vi "Set Comment.vi"(8 "error in (no error)":errorcluster, 10 "Comment":string, 11 "Device in":refnum<class "Device.lvclass">) -> (0 "error out":errorcluster, 3 "Device out":refnum<class "Device.lvclass">)   [LabVIEW 2012, in "HAL.lvlib" / "Device.lvclass"]
uses:
  Device.lvclass
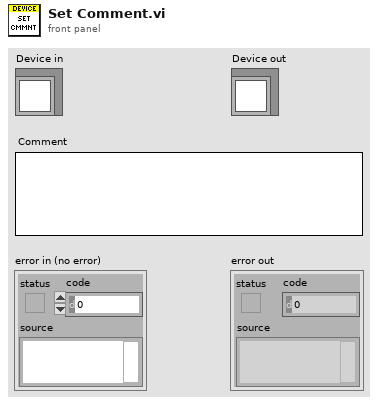
[diagram p1: front panel]
types:
  T1 = typedef "HAL.lvlib/Device.lvclass/Ref Data.ctl" = cluster{"Config Keys":string[], "Config Values":string[], "Cal Expires":timestamp, "Name":string, "Comment":string, "State":T2, "Error":errorcluster}
  T2 = typedef "HAL.lvlib/Device.lvclass/Device State.ctl" = enum16{"Uninitialized", "Initialized", "Ready", "Running", "Error"}
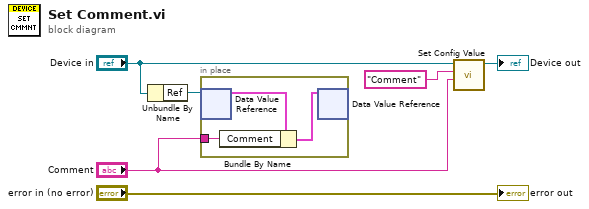
[diagram p0: block diagram]
diagram:
  n1 = Unbundle By Name("Device in") -> ("Ref"=w5:refnum<data-value>)
  n2 = in-place {
    in-place-border: "Comment" -> [w7]
    n3 = in-place-dvr #1(w5) -> (w9:T1)  [unwired: 1 out]
    n4 = Bundle By Name(cluster=w9, "Comment"=w7) -> (w8:T1)
    n5 = in-place-dvr #1(w8) -> ()  [unwired: 2 out]
  }
  n6 = call "Set Config Value.vi"("Value"="Comment", "Config Key"="Comment", "Device in"="Device in") -> ("Device out"=→"Device out":refnum<class "Device.lvclass">)  [unwired: 7 in, 1 out]
  "error out" <- "error in (no error)"
